vi "get_frame_rate.vi"(8 "error in (no error)":errorcluster, 11 "ImagingModeDL090130Frame in":refnum<class "ImagingModeDL090130Frame.lvclass">=refnum) -> (0 "error out":errorcluster, 2 "frame rate":dbl[unit], 3 "ImagingModeDL090130Frame out":refnum<class "ImagingModeDL090130Frame.lvclass">)   [LabVIEW 2010]
uses:
  ImagingModeDL090130Frame.lvclass
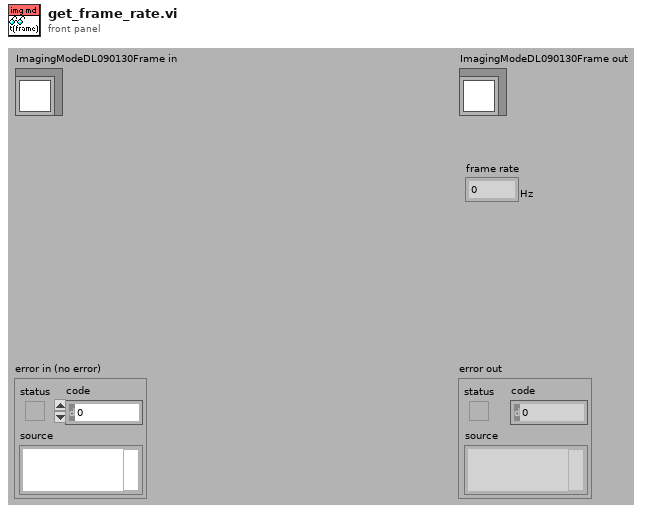
[diagram p1: front panel]
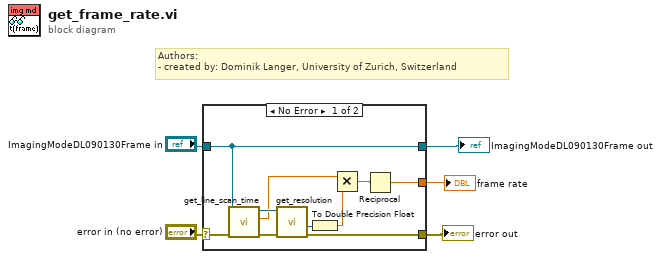
[diagram p0: block diagram]
diagram:
  # "Authors: \n- created by: Dominik Langer, University of Zurich, Switzerland"
  n1 = case shown="No Error" "error in (no error)" {
    selector: "error in (no error)" -> [w14 w17]
    tunnel: [w13 w17] -> w4
    tunnel: [w12 w16] -> w2
    tunnel: "ImagingModeDL090130Frame in" -> [w12 w16]
    tunnel: [w6 _] -> w1
    frame No Error {
      n2 = call-dynamic "get_line_scan_time.vi"("error in (no error)"=w14, "ImagingModeDL090130Frame in"=w12) -> ("error out"=w15:errorcluster, "line-scan time"=w10:dbl[unit], "ImagingModeDL090130Frame out"=w11:refnum<class "ImagingModeDL090130Frame.lvclass">)  [unwired: 7 out]
      n3 = call-dynamic "get_resolution.vi"("error in (no error)"=w15, "ImagingModeDL090130Frame in"=w11) -> ("error out"=w13:errorcluster, "y resolution"=w9:i32)  [unwired: 8 out]
      n4 = To Double Precision Float(number=w9) -> (double precision float=w8:dbl)
      n5 = Multiply(x=w10, y=w8) -> (x*y=w7:dbl[unit])
      n6 = Reciprocal(x=w7) -> (1/x=w6:dbl[unit])
    }
    frame Error {
    }
  }
  "error out" <- w4
  "ImagingModeDL090130Frame out" <- w2
  "frame rate" <- w1
